vi "demo - shift register while loop.vi"() -> ()   [LabVIEW 2024]
doc: "#vi_description \nPlot a sine wave onto a waveform chart with user adjustable wavelength. Historical plots are included.\nThetic Engineering Ltd."
panel:
  in  "Wavelength":u8(slide)=6 min=1 scale=1.0..10.0
  in  "Stop":bool
  out "Waveform Chart":cluster{dbl, dbl}(graph)
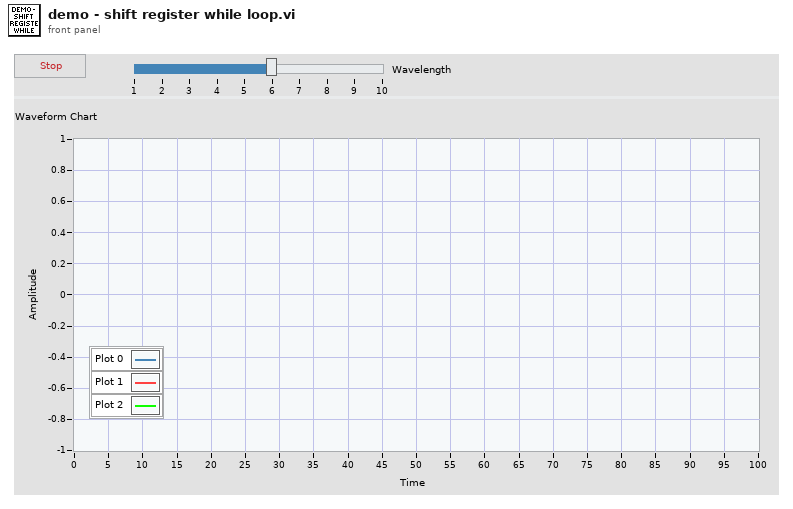
[diagram p1: front panel]
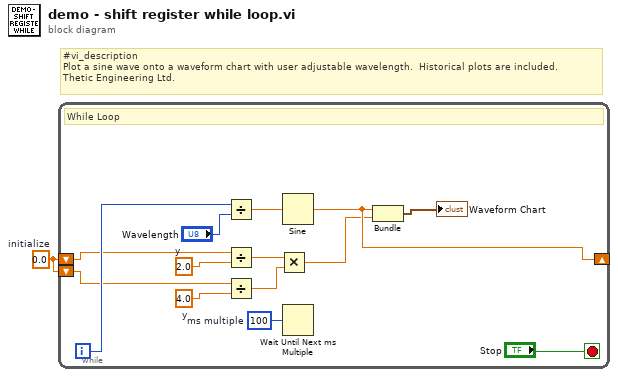
[diagram p0: block diagram]
diagram:
  w1 = 0.0  # initialize
  # "#vi_description \nPlot a sine wave onto a waveform chart with user adjustable wavelength.  Historical plots are included.\nThetic Engineering Ltd."
  n1 = while {
    shift-right: [w11] -> _
    shift-left: w1 -> [w9]
    shift-left: w1 -> [w8]
    i -> [w14]
    stop <- "Stop" stop-if-true
    w6 = 4.0  # y
    w7 = 2.0  # y
    w13 = u32 100  # ms multiple
    # "While Loop"
    n2 = Divide(x=w14, y="Wavelength") -> (x/y=w10:dbl)
    n3 = Divide(x=w9, y=w7) -> (x/y=w5:dbl)
    n4 = Divide(x=w8, y=w6) -> (x/y=w2:dbl)
    n5 = Multiply(x=w5, y=w2) -> (x*y=w3:dbl)
    n6 = Sine(x=w10) -> (sin(x)=w11:dbl)
    n7 = Wait Until Next ms Multiple(millisecond multiple=w13) -> ()  [unwired: 1 out]
    n8 = Bundle(w11, w3) -> (→"Waveform Chart":cluster{dbl, dbl})  [unwired: 1 in]
  }
